vi "OpenChannel2(SubVI).vi"(11 "VISA Refnum in":refnum<visa-resource-name>) -> ()   [LabVIEW 2022 SP3]
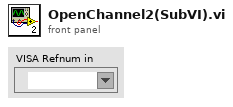
[diagram p1: front panel]
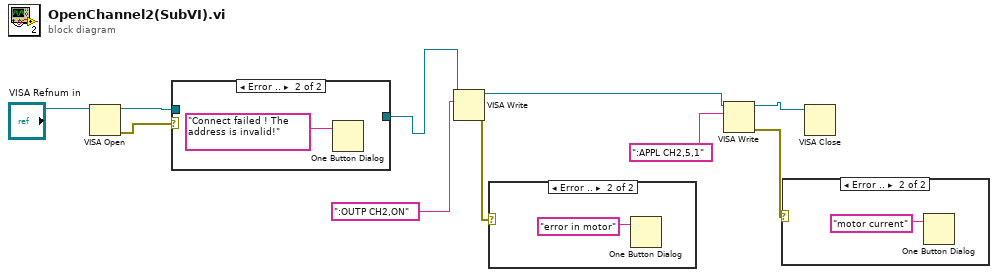
[diagram p0: block diagram]
diagram:
  n1 = VISA Open(VISA resource name="VISA Refnum in") -> (VISA resource name=w2:refnum<visa-resource-name>, error out=w3:errorcluster)  [unwired: 4 in]
  n2 = case shown="Error .." w3 {
    tunnel: w2 -> [w11 _]
    tunnel: [w11 _] -> w5
    frame No Error {
    }
    frame Error {
      n3 = One Button Dialog(message="Connect failed ! The address is invalid!") -> ()  [unwired: 1 in, 1 out]
    }
  }
  n4 = VISA Write(VISA resource name=w5, write buffer=":OUTP CH2,ON") -> (VISA resource name out=w8:refnum<visa-resource-name>, error out=w7:errorcluster)  [unwired: 1 in, 1 out]
  n5 = case shown="Error .." w7 {
    frame No Error {
    }
    frame Error {
      n6 = One Button Dialog(message="error in motor") -> ()  [unwired: 1 in, 1 out]
    }
  }
  n7 = VISA Write(VISA resource name=w8, write buffer=":APPL CH2,5,1") -> (VISA resource name out=w1:refnum<visa-resource-name>, error out=w10:errorcluster)  [unwired: 1 in, 1 out]
  n8 = case shown="Error .." w10 {
    frame No Error {
    }
    frame Error {
      n9 = One Button Dialog(message="motor current") -> ()  [unwired: 1 in, 1 out]
    }
  }
  n10 = VISA Close(VISA resource name=w1) -> ()  [unwired: 1 in, 1 out]
